vi "Rack-Stop.vi"(8 "error in (no error)":errorcluster, 11 "OutputRequest channel":T1) -> (0 "error out":errorcluster)   [LabVIEW 2015]
doc: "Stops the rack drivers running and releases any references.\n\nOutputRequest channel: User Event refnum for communicating with the output drivers."
uses:
  Typedefs/OutputRequest refnum.ctl
  Typedefs/OutputRequest.ctl
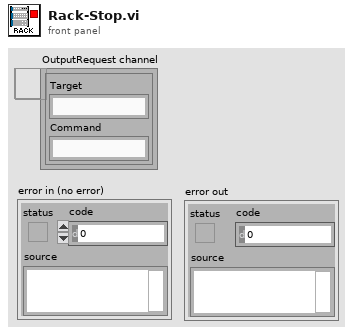
[diagram p1: front panel]
types:
  T1 = typedef "OutputRequest refnum.ctl" = refnum<user-event>
  T2 = typedef "OutputRequest.ctl" = cluster{"Target":string, "Command":string}
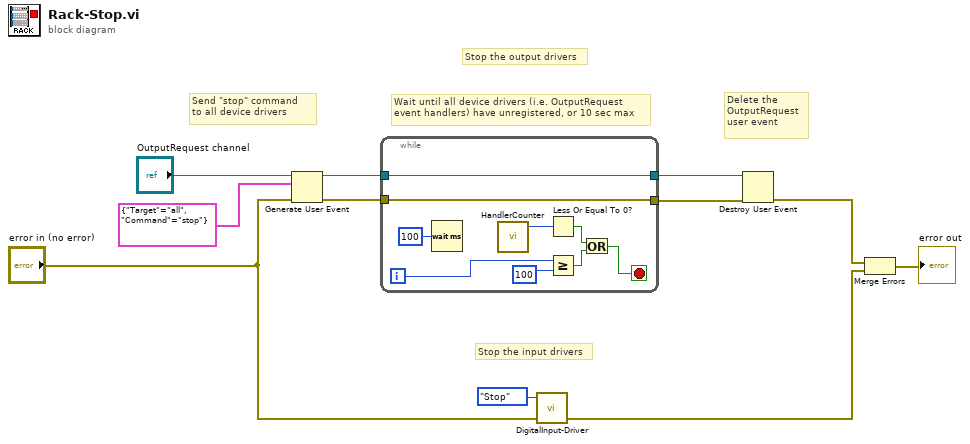
[diagram p0: block diagram]
diagram:
  # "Stop the input drivers"
  # "Stop the output drivers"
  # "Delete the \nOutputRequest\nuser event"
  # "Wait until all device drivers (i.e. OutputRequest\nevent handlers) have unregistered, or 10 sec max"
  # "Send \"stop\" command \nto all device drivers"
  n1 = Generate User Event(user event="OutputRequest channel", event data cluster=T2 {"Target"="all", "Command"="stop"} ("event data"), error in="error in (no error)") -> (user event out=w11:T1, error out=w10:errorcluster)  [unwired: 1 in]
  n2 = while {
    tunnel: [w18] -> w9
    tunnel: w11 -> [w18]
    tunnel: [w17] -> w8
    tunnel: w10 -> [w17]
    i -> [w16]
    stop <- w12 stop-if-true
    n3 = Wait (ms)(milliseconds to wait=u32 100) -> ()  [unwired: 1 out]
    n4 = call "HandlerCounter.vi"() -> ("Count"=w19:i16)  [unwired: 4 in, 1 out]
    n5 = Less Or Equal To 0?(x=w19) -> (x <= 0?=w13:bool)
    n6 = Greater Or Equal?(x=w16, y=100) -> (x >= y?=w14:bool)
    n7 = Or(x=w13, y=w14) -> (x .or. y?=w12:bool)
  }
  n8 = call "DigitalInput-Driver.vi"("error in (no error)"="error in (no error)", "Command"=enum16{"Refresh", "Start", "Stop"}."Stop") -> ("error out"=w2:errorcluster)  [unwired: 2 in, 1 out]
  n9 = Destroy User Event(user event=w9, error in=w8) -> (error out=w5:errorcluster)
  n10 = Merge Errors(w5, w2) -> (→"error out":errorcluster)
